vi "Smista DO.vi"(4 "Forza DO Cdaq":T4, 8 "Forza DO plc 3":T1, 9 "Forza DO plc 2":T2, 10 "Forza DO plc 1":T3, 11 "DO interfaccia in":T5) -> (0 "StatoDO_PLC_3_out":T1, 1 "StatoDO_PLC_2_out":T2, 2 "StatoDO_PLC_1_out":T3, 3 "statoDO Cdaq out":T4)   [LabVIEW 2019]
uses:
  cDAQ_PLC Folder/controls/statoDO_Cdaq.ctl
  cDAQ_PLC Folder/ST1200_LIST_IO/StatoDO_PLC_1.ctl
  TypeDef/DOinterfaccia.ctl
  cDAQ_PLC Folder/ST1200_LIST_IO/StatoDO_PLC_2.ctl
  cDAQ_PLC Folder/ST1200_LIST_IO/StatoDO_PLC_3.ctl
  GlobalForzaUscite.vi
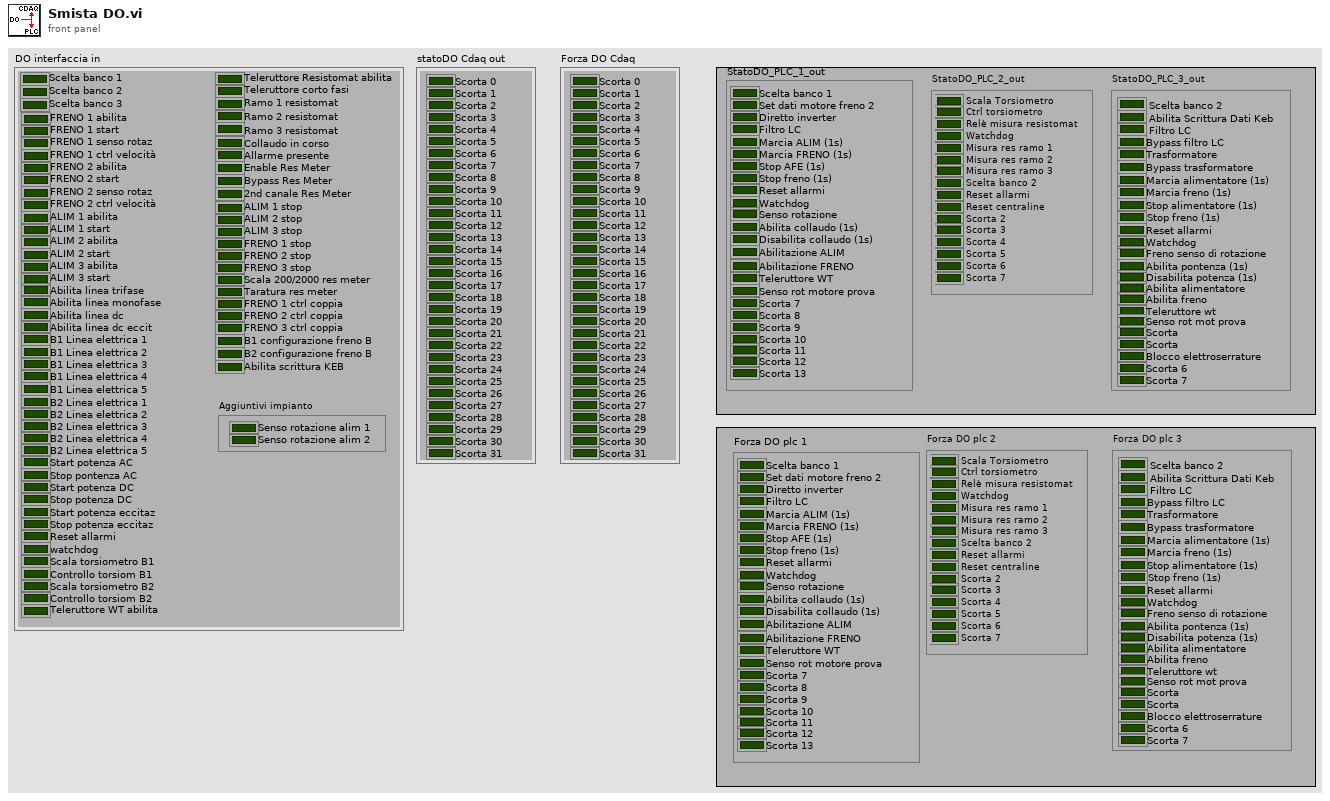
[diagram p1: front panel]
types:
  T1 = typedef "StatoDO_PLC_3.ctl" = cluster{"Scelta banco 2":bool, "Abilita Scrittura Dati Keb":bool, "Filtro LC":bool, "Bypass filtro LC":bool, "Trasformatore":bool, "Bypass trasformatore":bool, "Marcia alimentatore (1s)":bool, "Marcia freno (1s)":bool, "Stop alimentatore (1s)":bool, "Stop freno (1s)":bool, "Reset allarmi":bool, "Watchdog":bool, "Freno senso di rotazione":bool, "Abilita pontenza (1s)":bool, "Disabilita potenza (1s)":bool, "Abilita alimentatore":bool, "Abilita freno":bool, "Teleruttore wt":bool, "Senso rot mot prova":bool, "Scorta":bool, "Scorta":bool, "Blocco elettroserrature":bool, "Scorta 6":bool, "Scorta 7":bool}
  T2 = typedef "StatoDO_PLC_2.ctl" = cluster{"Scala Torsiometro":bool, "Ctrl torsiometro":bool, "Relè misura resistomat":bool, "Watchdog":bool, "Misura res ramo 1":bool, "Misura res ramo 2":bool, "Misura res ramo 3":bool, "Scelta banco 2":bool, "Reset allarmi":bool, "Reset centraline":bool, "Scorta 2":bool, "Scorta 3":bool, "Scorta 4":bool, "Scorta 5":bool, "Scorta 6":bool, "Scorta 7":bool}
  T3 = typedef "StatoDO_PLC_1.ctl" = cluster{"Scelta banco 1":bool, "Set dati motore freno 2":bool, "Diretto inverter":bool, "Filtro LC":bool, "Marcia ALIM (1s)":bool, "Marcia FRENO (1s)":bool, "Stop AFE (1s)":bool, "Stop freno (1s)":bool, "Reset allarmi":bool, "Watchdog":bool, "Senso rotazione":bool, "Abilita collaudo (1s)":bool, "Disabilita collaudo (1s)":bool, "Abilitazione ALIM":bool, "Abilitazione FRENO":bool, "Teleruttore WT":bool, "Senso rot motore prova":bool, "Scorta 7":bool, "Scorta 8":bool, "Scorta 9":bool, "Scorta 10":bool, "Scorta 11":bool, "Scorta 12":bool, "Scorta 13":bool}
  T4 = typedef "statoDO_Cdaq.ctl" = cluster{"Scorta 0":bool, "Scorta 1":bool, "Scorta 2":bool, "Scorta 3":bool, "Scorta 4":bool, "Scorta 5":bool, "Scorta 6":bool, "Scorta 7":bool, "Scorta 8":bool, "Scorta 9":bool, "Scorta 10":bool, "Scorta 11":bool, "Scorta 12":bool, "Scorta 13":bool, "Scorta 14":bool, "Scorta 15":bool, "Scorta 16":bool, "Scorta 17":bool, "Scorta 18":bool, "Scorta 19":bool, "Scorta 20":bool, "Scorta 21":bool, "Scorta 22":bool, "Scorta 23":bool, "Scorta 24":bool, "Scorta 25":bool, "Scorta 26":bool, "Scorta 27":bool, "Scorta 28":bool, "Scorta 29":bool, "Scorta 30":bool, "Scorta 31":bool}
  T5 = typedef "DOinterfaccia.ctl" = cluster{"Scelta banco 1":bool, "Scelta banco 2":bool, "Scelta banco 3":bool, "FRENO 1 abilita":bool, "FRENO 1 start":bool, "FRENO 1 senso rotaz":bool, "FRENO 1 ctrl velocità":bool, "FRENO 2 abilita":bool, "FRENO 2 start":bool, "FRENO 2 senso rotaz":bool, "FRENO 2 ctrl velocità":bool, "ALIM 1 abilita":bool, "ALIM 1 start":bool, "ALIM 2 abilita":bool, "ALIM 2 start":bool, "ALIM 3 abilita":bool, "ALIM 3 start":bool, "Abilita linea trifase":bool, "Abilita linea monofase":bool, "Abilita linea dc":bool, "Abilita linea dc eccit":bool, "B1 Linea elettrica 1":bool, "B1 Linea elettrica 2":bool, "B1 Linea elettrica 3":bool, "B1 Linea elettrica 4":bool, "B1 Linea elettrica 5":bool, "B2 Linea elettrica 1":bool, "B2 Linea elettrica 2":bool, "B2 Linea elettrica 3":bool, "B2 Linea elettrica 4":bool, "B2 Linea elettrica 5":bool, "Start potenza AC":bool, "Stop pontenza AC":bool, "Start potenza DC":bool, "Stop potenza DC":bool, "Start potenza eccitaz":bool, "Stop potenza eccitaz":bool, "Reset allarmi":bool, "watchdog":bool, "Scala torsiometro B1":bool, "Controllo torsiom B1":bool, "Scala torsiometro B2":bool, "Controllo torsiom B2":bool, "Teleruttore WT abilita":bool, "Teleruttore Resistomat abilita":bool, "Teleruttore corto fasi":bool, "Ramo 1 resistomat":bool, "Ramo 2 resistomat":bool, "Ramo 3 resistomat":bool, "Collaudo in corso":bool, "Allarme presente":bool, "Enable Res Meter":bool, "Bypass Res Meter":bool, "2nd canale Res Meter":bool, "Scala 200/2000 res meter":bool, "Taratura res meter":bool, "FRENO 1 ctrl coppia":bool, "FRENO 2 ctrl coppia":bool, "FRENO 3 ctrl coppia":bool, "Aggiuntivi impianto":cluster{"Senso rotazione alim 1":bool, "Senso rotazione alim 2":bool}, "ALIM 1 stop":bool, "ALIM 2 stop":bool, "ALIM 3 stop":bool, "FRENO 1 stop":bool, "FRENO 2 stop":bool, "FRENO 3 stop":bool, "B1 configurazione freno B":bool, "B2 configurazione freno B":bool, "Abilita scrittura KEB":bool}
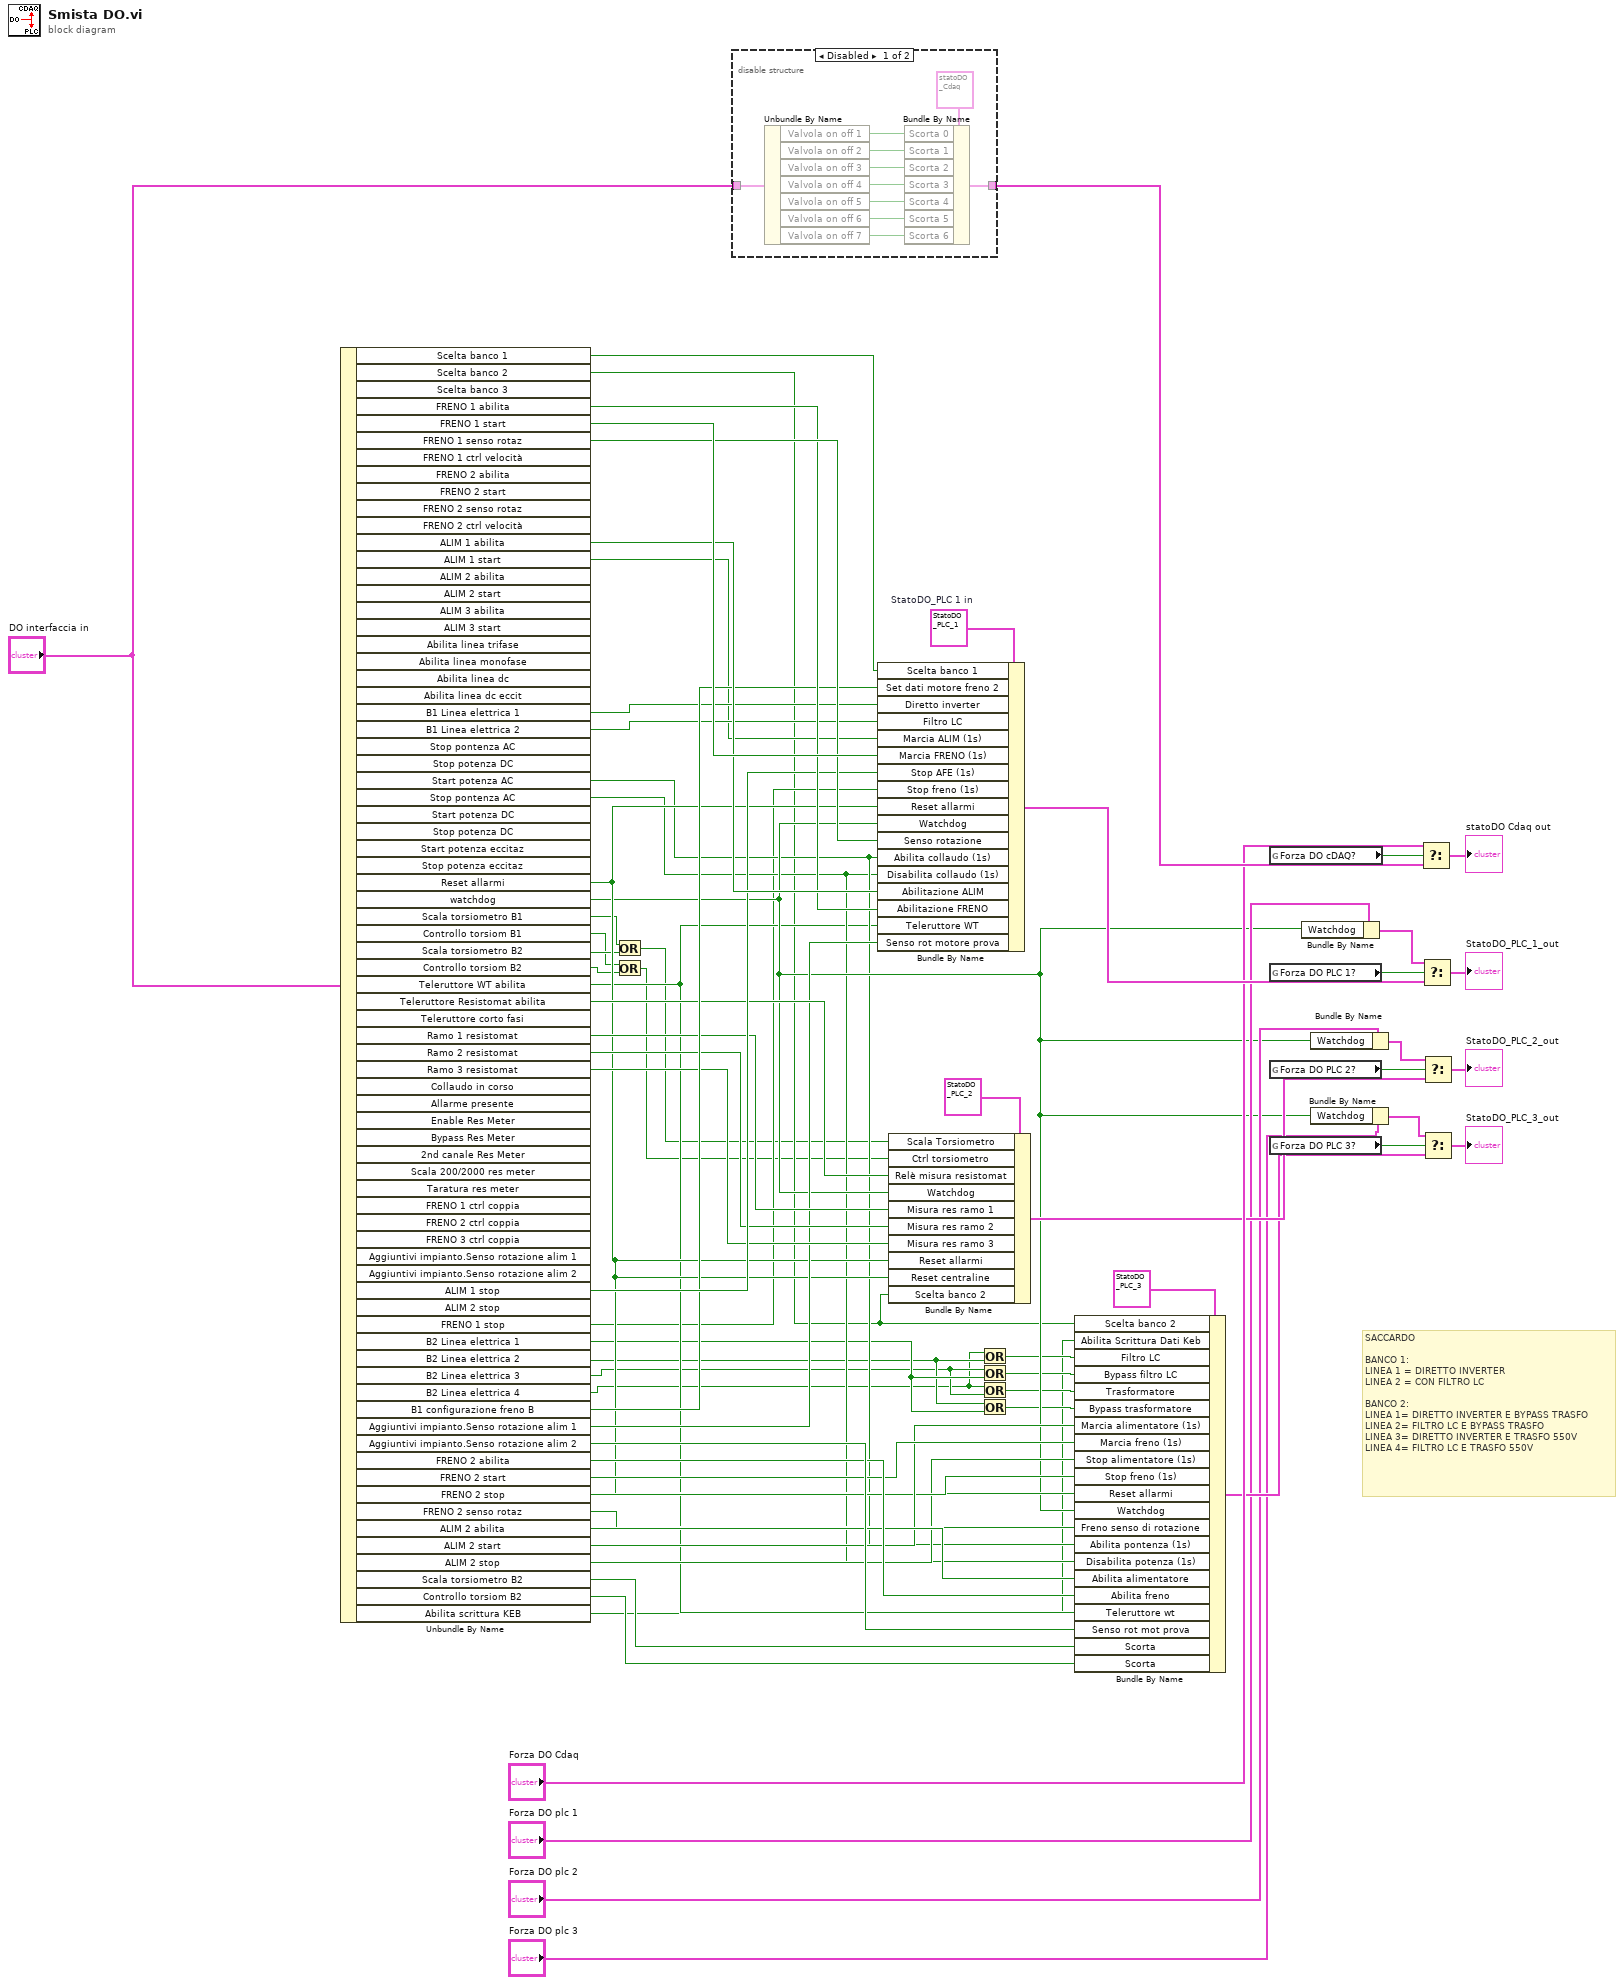
[diagram p0: block diagram]
diagram:
  w70 = T3 {"Scelta banco 1"=FALSE, "Set dati motore freno 2"=FALSE, "Diretto inverter"=FALSE, "Filtro LC"=FALSE, "Marcia ALIM (1s)"=FALSE, "Marcia FRENO (1s)"=FALSE, "Stop AFE (1s)"=FALSE, "Stop freno (1s)"=FALSE, "Reset allarmi"=FALSE, "Watchdog"=FALSE, "Senso rotazione"=FALSE, "Abilita collaudo (1s)"=FALSE, "Disabilita collaudo (1s)"=FALSE, "Abilitazione ALIM"=FALSE, "Abilitazione FRENO"=FALSE, "Teleruttore WT"=FALSE, "Senso rot motore prova"=FALSE, "Scorta 7"=FALSE, "Scorta 8"=FALSE, "Scorta 9"=FALSE, "Scorta 10"=FALSE, "Scorta 11"=FALSE, "Scorta 12"=FALSE, "Scorta 13"=FALSE}  # StatoDO_PLC 1 in
  # "SACCARDO\n\nBANCO 1:\nLINEA 1 = DIRETTO INVERTER\nLINEA 2 = CON FILTRO LC\n\nBANCO 2:\nLINEA 1= DIRETTO INVERTER E BYPASS TRASFO\nLINEA 2= FILTRO LC E BYPASS TRASFO\nLINEA 3= DIRETTO INVERTER E TRASFO 550V\nLINEA 4= FILTRO LC E TRASFO 550V"
  n1 = Unbundle By Name("DO interfaccia in") -> ("Scelta banco 1"=w18:bool, "Scelta banco 2"=w8:bool, "FRENO 1 abilita"=w46:bool, "FRENO 1 start"=w49:bool, "FRENO 1 senso rotaz"=w48:bool, "ALIM 1 abilita"=w47:bool, "ALIM 1 start"=w36:bool, "B1 Linea elettrica 1"=w43:bool, "B1 Linea elettrica 2"=w42:bool, "Start potenza AC"=w23:bool, "Stop pontenza AC"=w22:bool, "Reset allarmi"=w25:bool, "watchdog"=w24:bool, "Scala torsiometro B1"=w5:bool, "Controllo torsiom B1"=w3:bool, "Scala torsiometro B2"=w6:bool, "Controllo torsiom B2"=w2:bool, "Teleruttore WT abilita"=w21:bool, "Teleruttore Resistomat abilita"=w40:bool, "Ramo 1 resistomat"=w39:bool, "Ramo 2 resistomat"=w38:bool, "Ramo 3 resistomat"=w37:bool, "ALIM 1 stop"=w45:bool, "FRENO 1 stop"=w17:bool, "B2 Linea elettrica 1"=w15:bool, "B2 Linea elettrica 2"=w14:bool, "B2 Linea elettrica 3"=w13:bool, "B2 Linea elettrica 4"=w10:bool, "B1 configurazione freno B"=w44:bool, "Aggiuntivi impianto.Senso rotazione alim 1"=w35:bool, "Aggiuntivi impianto.Senso rotazione alim 2"=w33:bool, "FRENO 2 abilita"=w32:bool, "FRENO 2 start"=w31:bool, "FRENO 2 stop"=w27:bool, "FRENO 2 senso rotaz"=w28:bool, "ALIM 2 abilita"=w30:bool, "ALIM 2 start"=w29:bool, "ALIM 2 stop"=w26:bool, "Scala torsiometro B2"=w20:bool, "Controllo torsiom B2"=w19:bool, "Abilita scrittura KEB"=w7:bool)  [unwired: 34 out]
  n2 = Or(x=w5, y=w6) -> (x .or. y?=w4:bool)
  n3 = Or(x=w3, y=w2) -> (x .or. y?=w1:bool)
  n4 = disable-structure shown="Disabled" {
    disable-tunnel: [w79 _] -> w69
    disable-tunnel: "DO interfaccia in" -> [w78 _]
    frame Disabled {
      n5 = Unbundle By Name(w78) -> ("Valvola on off 1"=w77:bool, "Valvola on off 2"=w76:bool, "Valvola on off 3"=w75:bool, "Valvola on off 4"=w74:bool, "Valvola on off 5"=w73:bool, "Valvola on off 6"=w72:bool, "Valvola on off 7"=w71:bool)
      n6 = Bundle By Name(cluster=T4 {"Scorta 0"=FALSE, "Scorta 1"=FALSE, "Scorta 2"=FALSE, "Scorta 3"=FALSE, "Scorta 4"=FALSE, "Scorta 5"=FALSE, "Scorta 6"=FALSE, "Scorta 7"=FALSE, "Scorta 8"=FALSE, "Scorta 9"=FALSE, "Scorta 10"=FALSE, "Scorta 11"=FALSE, "Scorta 12"=FALSE, "Scorta 13"=FALSE, "Scorta 14"=FALSE, "Scorta 15"=FALSE, "Scorta 16"=FALSE, "Scorta 17"=FALSE, "Scorta 18"=FALSE, "Scorta 19"=FALSE, "Scorta 20"=FALSE, "Scorta 21"=FALSE, "Scorta 22"=FALSE, "Scorta 23"=FALSE, "Scorta 24"=FALSE, "Scorta 25"=FALSE, "Scorta 26"=FALSE, "Scorta 27"=FALSE, "Scorta 28"=FALSE, "Scorta 29"=FALSE, "Scorta 30"=FALSE, "Scorta 31"=FALSE} ("statoDO Cdaq in in"), "Scorta 0"=w77, "Scorta 1"=w76, "Scorta 2"=w75, "Scorta 3"=w74, "Scorta 4"=w73, "Scorta 5"=w72, "Scorta 6"=w71) -> (w79:T4)
    }
    frame Enabled {
    }
  }
  n7 = Bundle By Name(cluster=w70, "Scelta banco 1"=w18, "Set dati motore freno 2"=w44, "Diretto inverter"=w43, "Filtro LC"=w42, "Marcia ALIM (1s)"=w36, "Marcia FRENO (1s)"=w49, "Stop AFE (1s)"=w45, "Stop freno (1s)"=w17, "Reset allarmi"=w25, "Watchdog"=w24, "Senso rotazione"=w48, "Abilita collaudo (1s)"=w23, "Disabilita collaudo (1s)"=w22, "Abilitazione ALIM"=w47, "Abilitazione FRENO"=w46, "Teleruttore WT"=w21, "Senso rot motore prova"=w35) -> (w67:T3)
  n8 = Bundle By Name(cluster=T2 {"Scala Torsiometro"=FALSE, "Ctrl torsiometro"=FALSE, "Relè misura resistomat"=FALSE, "Watchdog"=FALSE, "Misura res ramo 1"=FALSE, "Misura res ramo 2"=FALSE, "Misura res ramo 3"=FALSE, "Scelta banco 2"=FALSE, "Reset allarmi"=FALSE, "Reset centraline"=FALSE, "Scorta 2"=FALSE, "Scorta 3"=FALSE, "Scorta 4"=FALSE, "Scorta 5"=FALSE, "Scorta 6"=FALSE, "Scorta 7"=FALSE} ("StatoDO_PLC_2_out"), "Scala Torsiometro"=w4, "Ctrl torsiometro"=w1, "Relè misura resistomat"=w40, "Watchdog"=w24, "Misura res ramo 1"=w39, "Misura res ramo 2"=w38, "Misura res ramo 3"=w37, "Reset allarmi"=w25, "Reset centraline"=w25, "Scelta banco 2"=w8) -> (w57:T2)
  n9 = Or(x=w10, y=w14) -> (x .or. y?=w12:bool)
  n10 = Or(x=w13, y=w15) -> (x .or. y?=w9:bool)
  n11 = Or(x=w10, y=w13) -> (x .or. y?=w11:bool)
  n12 = Or(x=w14, y=w15) -> (x .or. y?=w16:bool)
  n13 = Bundle By Name(cluster=T1 {"Scelta banco 2"=FALSE, "Abilita Scrittura Dati Keb"=FALSE, "Filtro LC"=FALSE, "Bypass filtro LC"=FALSE, "Trasformatore"=FALSE, "Bypass trasformatore"=FALSE, "Marcia alimentatore (1s)"=FALSE, "Marcia freno (1s)"=FALSE, "Stop alimentatore (1s)"=FALSE, "Stop freno (1s)"=FALSE, "Reset allarmi"=FALSE, "Watchdog"=FALSE, "Freno senso di rotazione"=FALSE, "Abilita pontenza (1s)"=FALSE, "Disabilita potenza (1s)"=FALSE, "Abilita alimentatore"=FALSE, "Abilita freno"=FALSE, "Teleruttore wt"=FALSE, "Senso rot mot prova"=FALSE, "Scorta"=FALSE, "Scorta"=FALSE, "Blocco elettroserrature"=FALSE, "Scorta 6"=FALSE, "Scorta 7"=FALSE} ("StatoDO_PLC_3_out"), "Scelta banco 2"=w8, "Abilita Scrittura Dati Keb"=w7, "Filtro LC"=w12, "Bypass filtro LC"=w9, "Trasformatore"=w11, "Bypass trasformatore"=w16, "Marcia alimentatore (1s)"=w29, "Marcia freno (1s)"=w31, "Stop alimentatore (1s)"=w26, "Stop freno (1s)"=w27, "Reset allarmi"=w25, "Watchdog"=w24, "Freno senso di rotazione"=w28, "Abilita pontenza (1s)"=w23, "Disabilita potenza (1s)"=w22, "Abilita alimentatore"=w30, "Abilita freno"=w32, "Teleruttore wt"=w21, "Senso rot mot prova"=w33, "Scorta"=w20, "Scorta"=w19) -> (w56:T1)
  n14 = global read "GlobalForzaUscite.vi" "Forza DO cDAQ?"() -> (w62:bool)
  n15 = global read "GlobalForzaUscite.vi" "Forza DO PLC 1?"() -> (w63:bool)
  n16 = global read "GlobalForzaUscite.vi" "Forza DO PLC 2?"() -> (w61:bool)
  n17 = global read "GlobalForzaUscite.vi" "Forza DO PLC 3?"() -> (w59:bool)
  n18 = Bundle By Name(cluster="Forza DO plc 1", "Watchdog"=w24) -> (w54:T3)
  n19 = Bundle By Name(cluster="Forza DO plc 2", "Watchdog"=w24) -> (w52:T2)
  n20 = Bundle By Name(cluster="Forza DO plc 3", "Watchdog"=w24) -> (w50:T1)
  n21 = Select(t="Forza DO Cdaq", s=w62, f=w69) -> (s? t:f=→"statoDO Cdaq out":T4)
  n22 = Select(t=w54, s=w63, f=w67) -> (s? t:f=→"StatoDO_PLC_1_out":T3)
  n23 = Select(t=w52, s=w61, f=w57) -> (s? t:f=→"StatoDO_PLC_2_out":T2)
  n24 = Select(t=w50, s=w59, f=w56) -> (s? t:f=→"StatoDO_PLC_3_out":T1)
